vi "cRIO9159_IO.vi"() -> ()   [LabVIEW 2013]
uses:
  datatypes/statesdaq.ctl
  <vilib>/rvi/Emulation/niFpgaSctlEmulationGetInTimedLoop.vi
  <vilib>/rvi/Emulation/niFpgaEmulationReportErrorSimple.vi
  <vilib>/rvi/Emulation/niFpgaGetClockAttributes.vi
  <vilib>/rvi/eio/common/nirviEmuTemplatePropertyGet_errors.vi
  <vilib>/rvi/eio/common/nirviEmuTemplateMethod_errors.vi
  <vilib>/rvi/Emulation/niFpgaCriticalErrorInLSC.vi
  <vilib>/eio/EIOPropertyNode/EIOPropertyNode.xnode
  <vilib>/eio/EIOMethodNode/EIOMethodNode.xnode
  <vilib>/eio/EIONode/EIONode.xnode
  <vilib>/rvi/eio/common/nirviEmuTemplatePropertyGet_noerrors.vi
  <vilib>/rvi/eio/common/nirviEmuTemplatePropertySet_errors.vi
  <vilib>/rvi/eio/common/nirviEmuTemplatePropertySet_noerrors.vi
panel:
  in  "Tab Control":T1(tab)=enum."Mandatory  Resources"
  out "Platform":enum8{"FlexRIO", "cRIO", "RSeries"}(ring)=enum."cRIO"
  out "FPGAVIversion":u8[](array[numeric])=[1, 1]
  out "InitDone":bool
  out "InsertedIOModulesID":u16[](array[numeric])
  out "cRIOModulesOK":bool
  out "Fref":u32=1000
  out "DevQualityStatus":u8
  out "DevTemp":i16=-3812
  out "DevProfile":u8=1
  in  "DAQStartStop":bool
  in  "DebugMode":bool
  in  "SamplingRate0":u16=1
  out "AI2":i32
  in  "AO2":i32
  out "AI0":i32
  out "AI1":i32
  out "auxAI0":i32
  out "auxAI1":i32
  in  "AO0":i32
  in  "AO1":i32
  in  "auxAO0":i32
  in  "auxAO1":i32
  in  "DO0":bool
  in  "DO1":bool
  out "DI0":bool
  out "DI1":bool
  in  "auxDO0":bool
  in  "auxDO1":bool
  out "auxDI0":bool
  out "auxDI1":bool
  out "SGNo":u8
  in  "AOEnable0":bool
  in  "AOEnable1":bool
  in  "AOEnable2":bool
  in  "DO2":bool
  out "DI2":bool
  out "state":T2=enum."acquisition"
  in  "Loop(uSec)":u32=1000 caption="Count(uSec)"
  # "fref should be greater then (1/N*4us)"
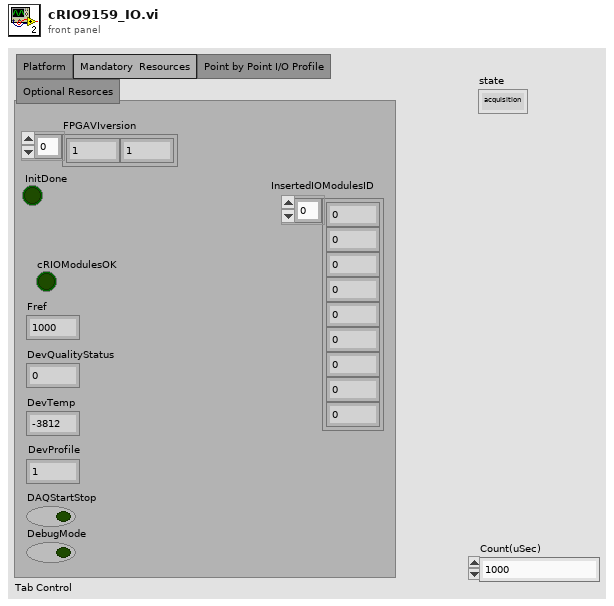
[diagram p1: front panel]
types:
  T1 = enum32{"Platform", "Mandatory  Resources", "Point by Point I/O Profile", "Optional Resorces"}
  T2 = typedef "statesdaq.ctl" = enum16{"init", "waitingtrigger", "acquisition", "error"}
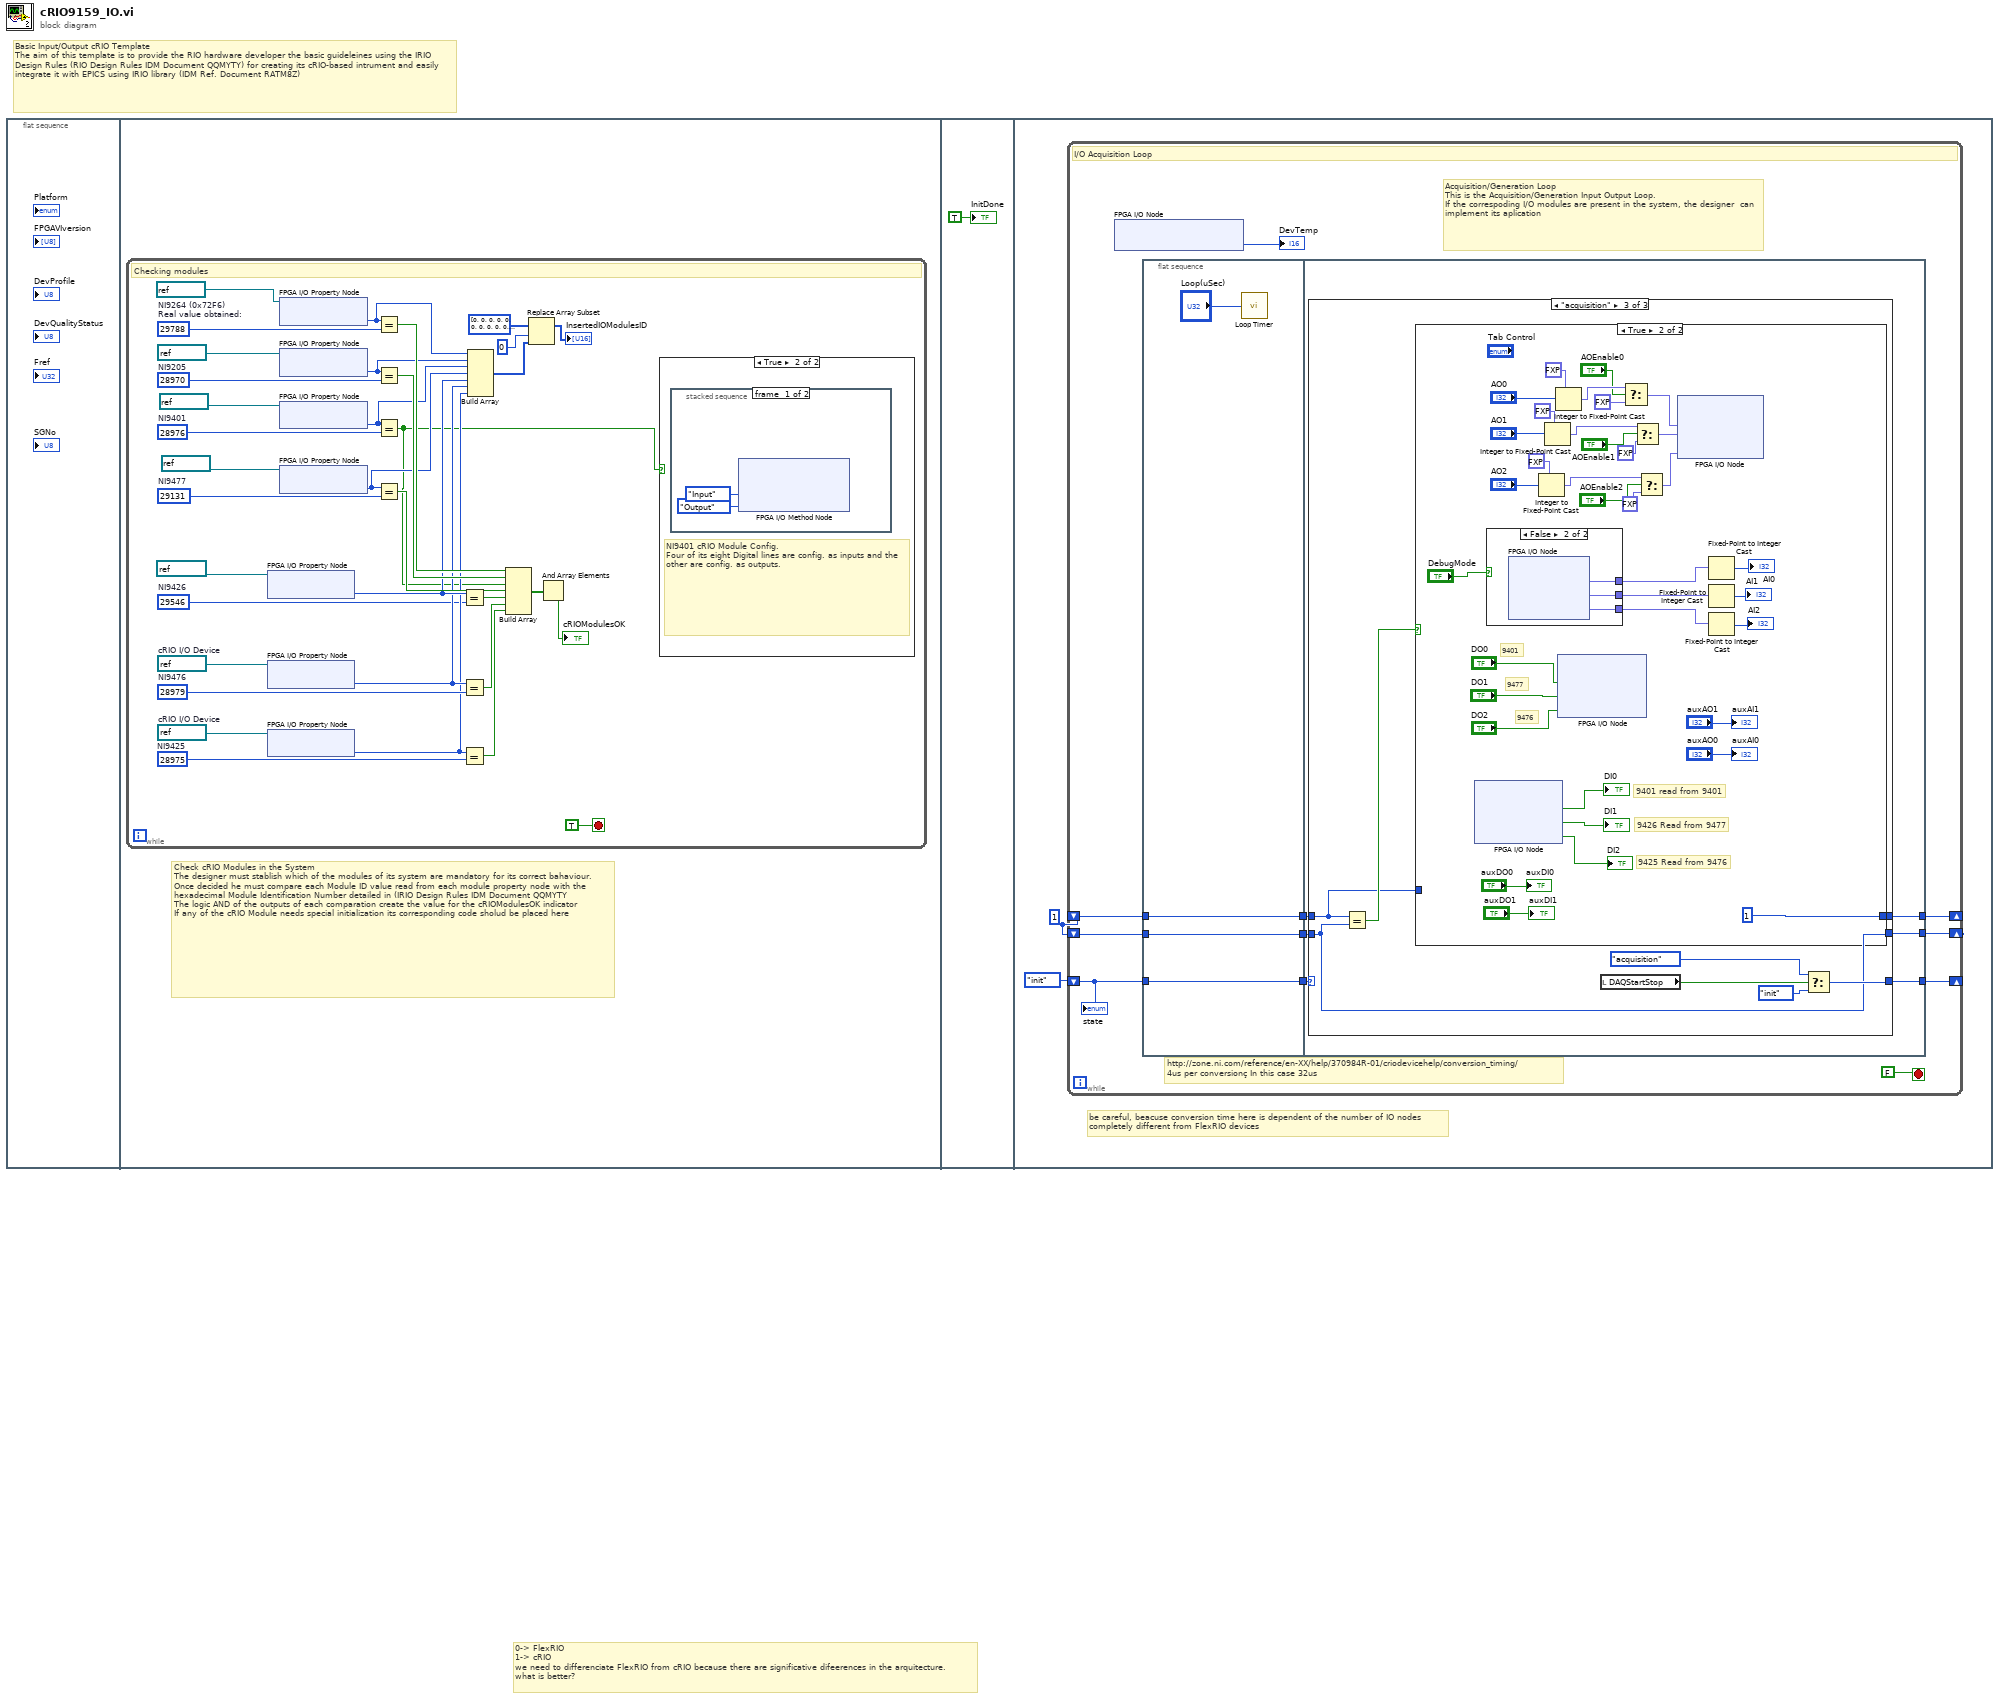
[diagram p0: block diagram]
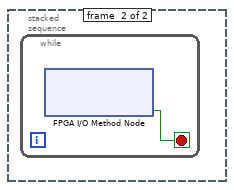
[diagram p3: hidden frame]
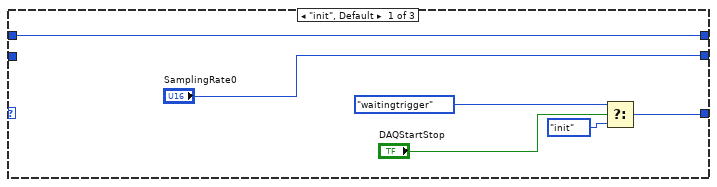
[diagram p4: hidden frame]
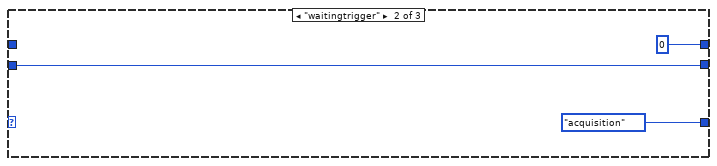
[diagram p5: hidden frame]
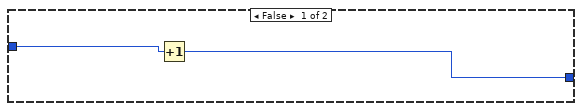
[diagram p6: hidden frame]
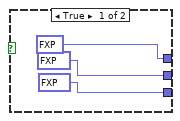
[diagram p7: hidden frame]
diagram:
  # "Basic Input/Output cRIO Template\nThe aim of this template is to provide the RIO hardware developer the basic guideleines using the IRIO Design Rules (RIO Design Rules IDM Document QQMYTY) for creating its cRIO-based intrument and easily integrate it with EPICS using IRIO library (IDM Ref. Document RATM8Z)"
  # "0-> FlexRIO\n1-> cRIO\nwe need to differenciate FlexRIO from cRIO because there are significative difeerences in the arquitecture.\nwhat is better?"
  n1 = flat-sequence {
    frame #0 {
    }
    frame #1 {
      # "Check cRIO Modules in the System\nThe designer must stablish which of the modules of its system are mandatory for its correct bahaviour. \nOnce decided he must compare each Module ID value read from each module property node with the hexadecimal Module Identification Number detailed in (IRIO Design Rules IDM Document QQMYTY\nThe logic AND of the outputs of each comparation create the value for the cRIOModulesOK indicator\nIf any of the cRIO Module needs special initialization its corresponding code sholud be placed here"
      n2 = while {
        stop <- TRUE stop-if-true
        w9 = u16 28975  # NI9425
        w10 = u16 29546  # NI9426
        w12 = u16 29131  # NI9477
        w14 = u16 28976  # NI9401
        w15 = u16 28970  # NI9205
        w13 = u16 29788  # NI9264 (0x72F6)  Real value obtained:
        w17 = refnum<k21> "Mod7"  # cRIO I/O Device
        w18 = refnum<k21> "Mod6"  # cRIO I/O Device
        w28 = u16 28979  # NI9476
        # "Checking modules"
        n3 = xnode "FPGA I/O Property Node"("FPGA I/O In"=refnum<k21> "Mod5") -> ("Module ID"=w23:u16)  [unwired: 1 in, 2 out]
        n4 = xnode "FPGA I/O Property Node"("FPGA I/O In"=w18) -> ("Module ID"=w22:u16)  [unwired: 1 in, 2 out]
        n5 = xnode "FPGA I/O Property Node"("FPGA I/O In"=w17) -> ("Module ID"=w21:u16)  [unwired: 1 in, 2 out]
        n6 = xnode "FPGA I/O Property Node"("FPGA I/O In"=refnum<k21> "Mod1") -> ("Module ID"=w2:u16)  [unwired: 1 in, 2 out]
        n7 = xnode "FPGA I/O Property Node"("FPGA I/O In"=refnum<k21> "Mod2") -> ("Module ID"=w24:u16)  [unwired: 1 in, 2 out]
        n8 = xnode "FPGA I/O Property Node"("FPGA I/O In"=refnum<k21> "Mod3") -> ("Module ID"=w3:u16)  [unwired: 1 in, 2 out]
        n9 = xnode "FPGA I/O Property Node"("FPGA I/O In"=refnum<k21> "Mod4") -> ("Module ID"=w11:u16)  [unwired: 1 in, 2 out]
        n10 = Equal?(x=w2, y=w13) -> (x = y?=w35:bool)
        n11 = Equal?(x=w24, y=w15) -> (x = y?=w34:bool)
        n12 = Equal?(x=w3, y=w14) -> (x = y?=w4:bool)
        n13 = Equal?(x=w11, y=w12) -> (x = y?=w33:bool)
        n14 = Equal?(x=w23, y=w10) -> (x = y?=w32:bool)
        n15 = Equal?(x=w22, y=w28) -> (x = y?=w31:bool)
        n16 = Equal?(x=w21, y=w9) -> (x = y?=w30:bool)
        n17 = Build Array(w2, w24, w3, w11, w23, w22, w21) -> (w20:u16[])
        n18 = Build Array(w35, w34, w4, w33, w32, w31, w30) -> (w29:bool[])
        n19 = Replace Array Subset(array=u16[] [0, 0, 0, 0, 0, 0, 0, 0, 0, 0, 0, 0, 0, 0, 0, 0] ("InsertedIOModulesID"), new element=w20, index=0) -> (→"InsertedIOModulesID":u16[])
        n20 = And Array Elements(Boolean array=w29) -> (logical AND=→"cRIOModulesOK":bool)
        n21 = case shown="True" w4 {
          frame False {
          }
          frame True {
            # "NI9401 cRIO Module Config.\nFour of its eight Digital lines are config. as inputs and the other are config. as outputs."
            n22 = stacked-sequence {
              frame #0 {
                n23 = xnode "FPGA I/O Method Node"("DIO 7:4"=enum8{"No Change", "Input", "Output"}."Input", "DIO 3:0"=enum8{"No Change", "Input", "Output"}."Output") -> ()  [unwired: 2 in, 2 out]
              }
              frame #1 {
                n24 = while {
                  stop <- w38 stop-if-true
                  n25 = xnode "FPGA I/O Method Node"() -> ("Ready"=w38:bool)  [unwired: 1 in, 1 out]
                }
              }
            }
          }
        }
      }
    }
    frame #2 {
      "InitDone" <- TRUE ("InitDone")
    }
    frame #3 {
      w40 = u16 1
      # "be careful, beacuse conversion time here is dependent of the number of IO nodes\ncompletely different from FlexRIO devices"
      n26 = while {
        shift-right: [w49] -> _
        shift-left: statesdaq."init" -> [w50]
        shift-right: [w47] -> _
        shift-left: w40 -> [w45]
        shift-right: [w44] -> _
        shift-left: w40 -> [w42]
        stop <- FALSE stop-if-true
        # "Acquisition/Generation Loop\nThis is the Acquisition/Generation Input Output Loop.\nIf the correspoding I/O modules are present in the system, the designer  can implement its aplication"
        # "http://zone.ni.com/reference/en-XX/help/370984R-01/criodevicehelp/conversion_timing/\n4us per conversionç In this case 32us"
        # "I/O Acquisition Loop"
        n27 = xnode "FPGA I/O Node"() -> ("Chassis Temperature"=→"DevTemp":i16)  [unwired: 1 in, 1 out]
        n28 = flat-sequence {
          tunnel: [w55] -> w51
          tunnel: w50 -> [w55]
          tunnel: [w54] -> w46
          tunnel: w45 -> [w54]
          tunnel: [w53] -> w43
          tunnel: w42 -> [w53]
          tunnel: w51 -> [w62]
          tunnel: [w61] -> w49
          tunnel: [w60] -> w47
          tunnel: w46 -> [w59]
          tunnel: [w58] -> w44
          tunnel: w43 -> [w57]
          frame #0 {
            n29 = call "Loop Timer"("Count(uSec)"="Loop(uSec)") -> ()  [unwired: 1 out]
          }
          frame #1 {
            n30 = case shown="\"acquisition\"" w62 {
              tunnel: [w65 statesdaq."acquisition" w76] -> w61
              tunnel: [w64 i16 0 w75] -> w60
              tunnel: w59 -> [w64 _ w73]
              tunnel: ["SamplingRate0" w69 w72] -> w58
              tunnel: w57 -> [_ w69 w72]
              frame "init", Default {
                n31 = Select(t=statesdaq."waitingtrigger", s="DAQStartStop", f=statesdaq."init") -> (s? t:f=w65:T2)
              }
              frame "waitingtrigger" {
              }
              frame "acquisition" {
                n32 = Equal?(x=w73, y=w72) -> (x = y?=w74:bool)
                n33 = case shown="True" w74 {
                  tunnel: [w81 u16 1] -> w75
                  tunnel: w73 -> [w80 _]
                  frame False {
                    n34 = Increment(x=w80) -> (x+1=w81:u16)
                  }
                  frame True {
                    # "9425 Read from 9476"
                    # "9426 Read from 9477"
                    # "9401 read from 9401"
                    # "9476"
                    # "9477"
                    # "9401"
                    n35 = xnode "FPGA I/O Node"() -> ("Mod3/DIO4"=→"DI0":bool, "Mod5/DI0"=→"DI1":bool, "Mod7/DI0"=→"DI2":bool)  [unwired: 4 in, 4 out]
                    n36 = case shown="False" "DebugMode" {
                      tunnel: [fxp<+/-,26,5> 1.25 ("fixed-point") w123] -> w105
                      tunnel: [fxp<+/-,26,5> -4.75 ("fixed-point") w122] -> w103
                      tunnel: [fxp<+/-,26,5> 3.125 ("fixed-point") w121] -> w102
                      frame True {
                      }
                      frame False {
                        n37 = xnode "FPGA I/O Node"() -> ("Mod2/AI0"=w123:fxp<+/-,26,5>, "Mod2/AI1"=w121:fxp<+/-,26,5>, "Mod2/AI2"=w122:fxp<+/-,26,5>)  [unwired: 4 in, 4 out]
                      }
                    }
                    n38 = Integer to Fixed-Point Cast(fixed-point type=fxp<+/-,20,5> 0.0 ("Mod4/AO0"), integer="AO2") -> (fixed-point=w85:fxp<+/-,20,5>)
                    n39 = Integer to Fixed-Point Cast(fixed-point type=fxp<+/-,20,5> 0.0 ("Mod4/AO0"), integer="AO1") -> (fixed-point=w89:fxp<+/-,20,5>)
                    n40 = Integer to Fixed-Point Cast(fixed-point type=fxp<+/-,20,5> 0.0 ("Mod4/AO0"), integer="AO0") -> (fixed-point=w96:fxp<+/-,20,5>)
                    n41 = xnode "FPGA I/O Node"("Mod3/DIO0"="DO0", "Mod4/DO0"="DO1", "Mod6/DO0"="DO2") -> ()  [unwired: 4 in, 4 out]
                    n42 = Select(t=w96, s="AOEnable0", f=fxp<+/-,20,5> 0.0) -> (s? t:f=w95:fxp<+/-,20,5>)
                    n43 = Select(t=w89, s="AOEnable1", f=fxp<+/-,20,5> 0.0) -> (s? t:f=w90:fxp<+/-,20,5>)
                    n44 = Select(t=w85, s="AOEnable2", f=fxp<+/-,20,5> 0.0) -> (s? t:f=w87:fxp<+/-,20,5>)
                    n45 = xnode "FPGA I/O Node"("Mod1/AO0"=w95, "Mod1/AO1"=w90, "Mod1/AO2"=w87) -> ()  [unwired: 4 in, 4 out]
                    n46 = Fixed-Point to Integer Cast(1:w105) -> (0:→"AI0":i32)
                    n47 = Fixed-Point to Integer Cast(1:w102) -> (0:→"AI1":i32)
                    n48 = Fixed-Point to Integer Cast(1:w103) -> (0:→"AI2":i32)
                    "auxAI0" <- "auxAO0"
                    "auxAI1" <- "auxAO1"
                    "auxDI0" <- "auxDO0"
                    "auxDI1" <- "auxDO1"
                  }
                }
                n49 = local read "DAQStartStop"() -> (w79:bool)
                n50 = Select(t=statesdaq."acquisition", s=w79, f=statesdaq."init") -> (s? t:f=w76:T2)
              }
            }
          }
        }
        "state" <- w50
      }
    }
  }
